vi "Fluigent_Pressure_Fluctuation_v3.vi"() -> ()   [LabVIEW 2020]
uses:
  <vilib>/DAQmx/read.llb/DAQmx Read (Analog 1D Wfm NChan NSamp).vi
  <userlib>/Fluigent/Fluigent MFCS/FluigentMFCS_Full.llb/MFCS_EZ Detect.vi
  <userlib>/Fluigent/Fluigent MFCS/FluigentMFCS_Full.llb/MFCS_EZ Initialization.vi
  <vilib>/DAQmx/create/channels.llb/DAQmx Create Channel (AI-Voltage-Basic).vi
  <vilib>/DAQmx/configure/timing.llb/DAQmx Timing (Sample Clock).vi
  <vilib>/DAQmx/miscellaneous.llb/DAQmx Fill In Error Info.vi
  <vilib>/Waveform/WDTOps.llb/WDT Get XY Value DBL.vi
  <userlib>/Fluigent/Fluigent MFCS/FluigentMFCS_Full.llb/MFCS_EZ Read All Channels Pressure.vi
  <userlib>/Fluigent/Fluigent MFCS/FluigentMFCS_Full.llb/MFCS_EZ Close.vi
  <vilib>/measure/NI_MABase.lvlib
panel:
  in  "Voltage Conversion Factor":dbl=100.0 caption="Voltage Conversion Factor (1 V = x mmHg)" format="%0.2f"
  out "Finished":bool
  out "Time Elapsed (Min)":cluster{dbl, dbl}(slide)={5.0, 0.0} scale=0.0..5.0 scale format="%#_2g"
  out "Dev1 Samples":i32
  out "Running":bool
  in  "sampling info":cluster{"Fs":dbl, "#s":dbl}
  in  "Fs":dbl
  in  "Time (min)":dbl(knob)=5.0 min=0.1 max=5.0 step=0.1 scale=0.0..5.0 scale format="%#_2g"
  in  "Index File Labels Fluigent System":string[](array[string])=["1000", "nobody", "test", "1", "1", "junk"]
  out "Analog File Name Fluigent":string="C:\\yurong\\141104_12_31_1104"
  in  "Path for files Fluigent System":path=path "C:/Users/kkg5246/Desktop/Research/Fluigent Recordings"
  out "Current Voltage (V)":dbl
  out "Current Pressure (mmHg)":dbl
  out "Actual Pressure":dbl[](graph)
  out "Theoretical Pressure Waveform":waveform(dbl)(graph)={"t0"=timestamp(15 s since 1904-01-01), "dt"=0.001, "Y"=[]}
  in  "Duty Cycle (%)":dbl=50.0 format="%0.2f"
  in  "Offset":dbl=250.0 format="%0.2p"
  in  "Reset Signal ?":bool
  in  "Signal Type":T1(ring)
  in  "Frequency (Hz)":dbl=5.0 format="%0.2p"
  in  "Amplitude (mmHg)":dbl=0.25 format="%0.2p"
  in  "Phase":dbl format="%0.2f"
  out "Phase out":dbl=180.0000000002135 format="%0.2f"
  in  "Stop":bool
  out "Waveform Chart":waveform(dbl)(graph)
  out "Pressure":dbl[](graph)=[0.00694105110600887]
  in  "physical channels":tag="Dev1/ai0"
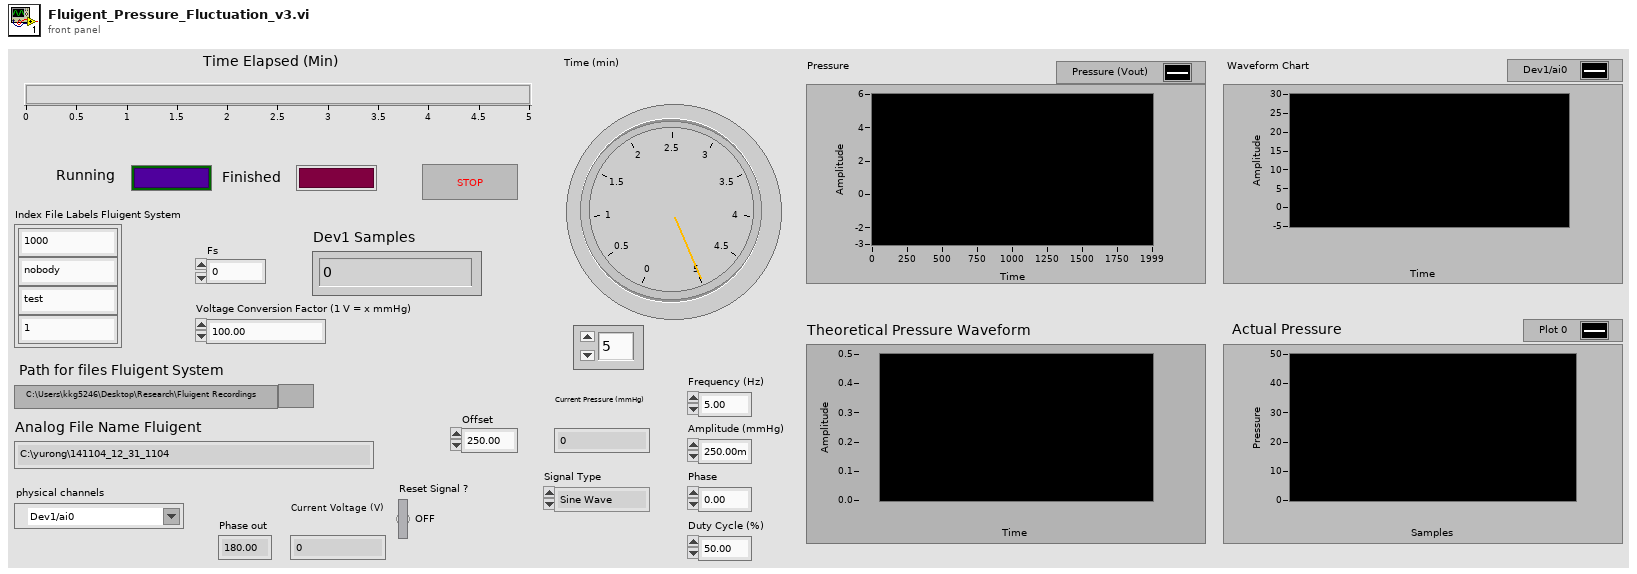
[diagram p1: front panel]
types:
  T1 = enum16{"Sine Wave", "Triangle Wave", "Square Wave", "Sawtooth Wave"}
  T2 = enum16{"open", "open or create", "create or replace", "create", "open (read-only)"}
  T3 = typedef "_EZmfcsSN.ctl" = u16
  T4 = typedef "_mfcs_EZ_handle.ctl" = u64
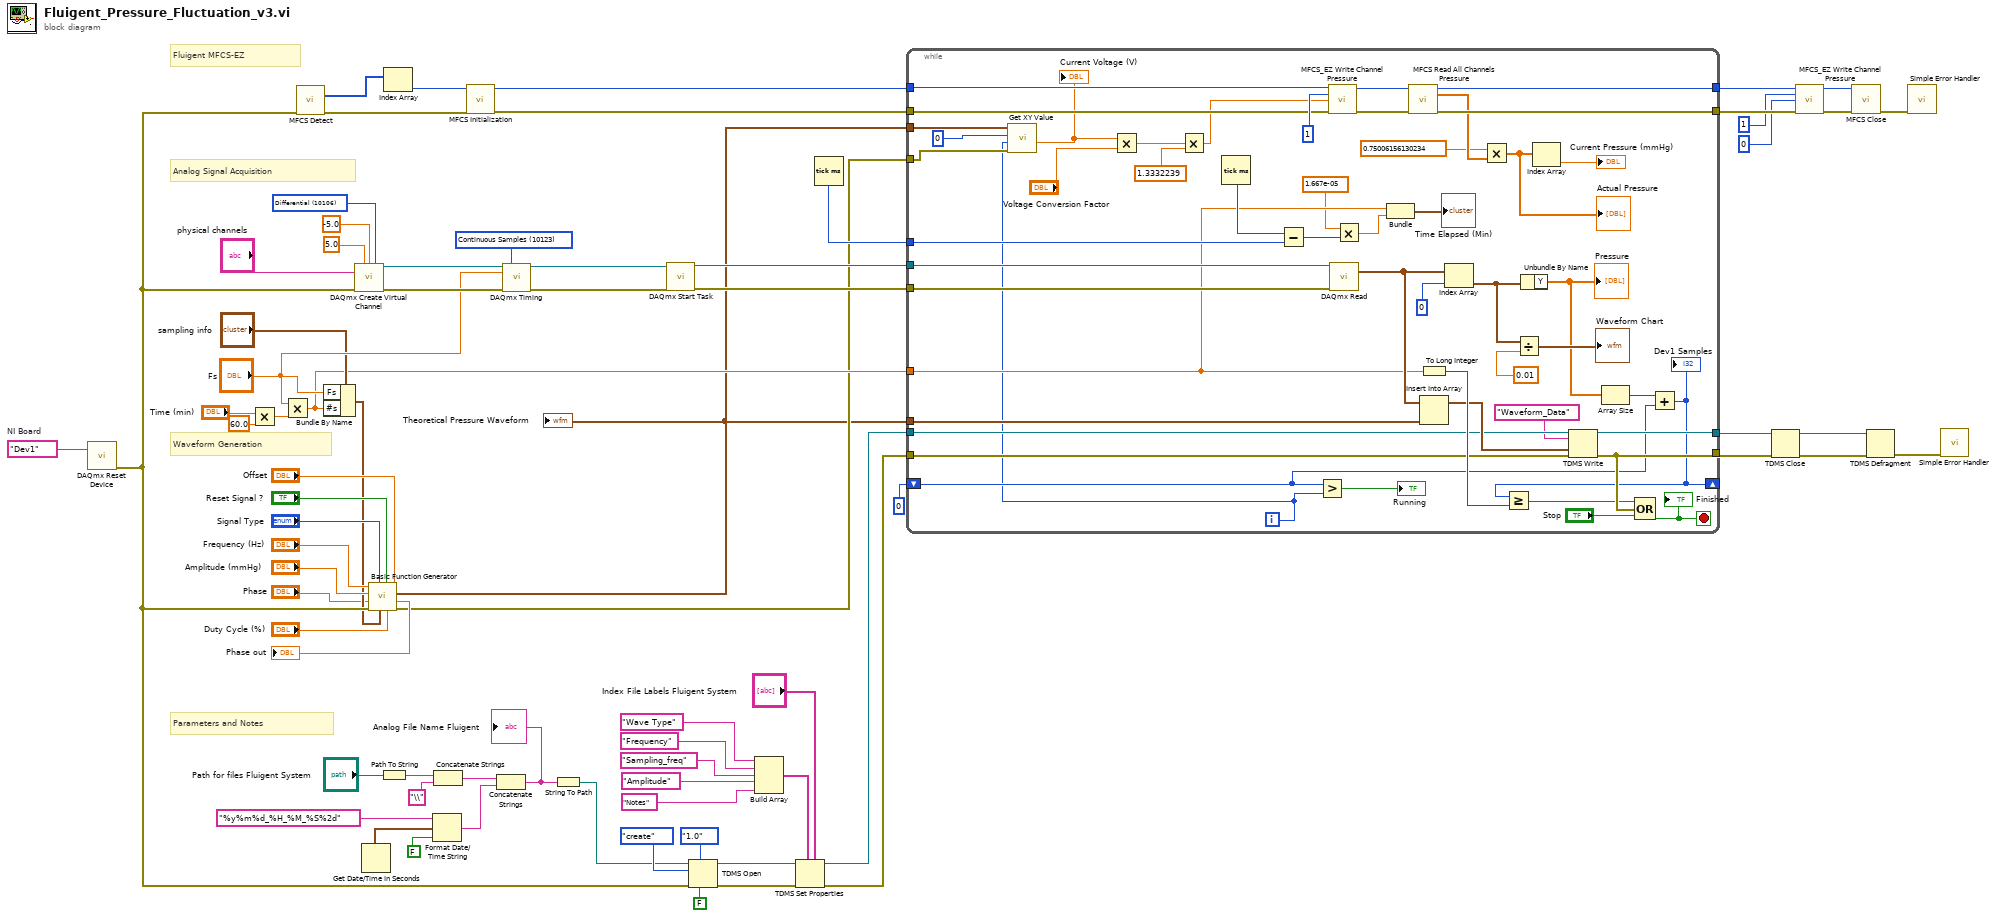
[diagram p0: block diagram]
diagram:
  w17 = tag "Dev1"  # NI Board
  w68 = 10106 items=["default"=-1, "RSE"=10083, "NRSE"=10078, "Differential"=10106, "Pseudodifferential"=12529] ("input terminal configuration")
  w72 = 10123 items=["Finite Samples"=10178, "Continuous Samples"=10123, "Hardware Timed Single Point"=12522] ("sample mode")
  # "Parameters and Notes"
  # "Waveform Generation"
  # "Analog Signal Acquisition"
  # "Fluigent MFCS-EZ"
  n1 = call <vilib>:"DAQmx Reset Device.vi"("device in"=w17) -> ("error out"=w16:errorcluster)  [unwired: 14 in]
  n2 = Multiply(x="Time (min)", y=60.0 ("minimum value")) -> (x*y=w5:dbl)
  n3 = Multiply(x="Fs", y=w5) -> (x*y=w9:dbl)
  n4 = call-poly <userlib>:"MFCS Detect.vi"("error in (no error)"=w16) -> ("[SN MFCS_EZ]"=w62:T3[], "error out"=w60:errorcluster)  [unwired: 13 in]
  n5 = Bundle By Name ("sampling info")(cluster="sampling info", "Fs"="Fs", "#s"=w9) -> (w15:cluster{"Fs":dbl, "#s":dbl})
  n6 = call-poly <vilib>:"DAQmx Create Virtual Channel.vi"("maximum value"=5.0, "minimum value"=-5.0, "input terminal configuration"=w68, "physical channels"="physical channels", "error in"=w16) -> ("task out"=w73:refnum<k21>, "error out"=w71:errorcluster)  [unwired: 4 in, 5 out]
  n7 = Get Date/Time In Seconds() -> (seconds since 1Jan1904=w48:timestamp)
  n8 = call <vilib>:"Basic Function Generator.vi"("offset"="Offset", "square wave duty cycle (%)"="Duty Cycle (%)", "reset signal"="Reset Signal ?", "sampling info"=w15, "signal type"="Signal Type", "error in (no error)"=w16, "phase"="Phase", "amplitude"="Amplitude (mmHg)", "frequency"="Frequency (Hz)") -> ("error out"=w2:errorcluster, "phase out"=→"Phase out":dbl, "signal out"=w1:waveform(dbl))
  "Theoretical Pressure Waveform" <- w1
  n9 = Path To String(path="Path for files Fluigent System") -> (string=w33:string)
  n10 = Index Array(array=w62) -> (element=w61:T3)  [unwired: 1 in]
  n11 = Format Date/Time String(time format string (%c)="%y%m%d_%H_%M_%S%2d", seconds (now)=w48, UTC format=FALSE) -> (date/time string=w45:string)
  n12 = Concatenate Strings(w33, "\\" ("string")) -> (w46:string)
  n13 = call-poly <userlib>:"MFCS Initialization.vi"("SN MFCS_EZ"=w61, "error in (no error)"=w60) -> ("MFCS_EZ_out"=w56:T4, "error out"=w55:errorcluster)  [unwired: 10 in, 2 out]
  n14 = Concatenate Strings(w46, w45) -> (w44:string)
  "Analog File Name Fluigent" <- w44
  n15 = call-poly <vilib>:"DAQmx Timing.vi"("task/channels in"=w73, "sample mode"=w72, "rate"="Fs", "error in"=w71) -> ("task out"=w66:refnum<k21>, "error out"=w65:errorcluster)  [unwired: 3 in, 7 out]
  n16 = String To Path(string=w44) -> (path=w40:path)
  n17 = call <vilib>:"DAQmx Start Task.vi"("task/channels in"=w66, "error in"=w65) -> ("task out"=w64:refnum<k21>, "error out"=w63:errorcluster)  [unwired: 12 out]
  n18 = TDMS Open(6:FALSE ("disable buffering? (T)"), 7:enum16{"1.0", "2.0"}."1.0" ("file format version (2.0)"), 8:w16, 10:T2."create" ("operation (0:open)"), 11:w40) -> (0:w39:errorcluster, 3:w31:refnum<k34>)  [unwired: 2 in]
  n19 = Build Array("Wave Type", "Frequency", "Sampling_freq", "Amplitude", "Notes") -> (w34:string[])
  n20 = TDMS Set Properties(5:"Index File Labels Fluigent System", 7:w34, 8:w39, 11:w31) -> (0:w29:errorcluster, 3:w26:refnum<k34>)  [unwired: 4 out]
  n21 = Tick Count (ms)() -> (millisecond timer value=w6:u32)
  n22 = while {
    tunnel: w64 -> [w119]
    tunnel: w63 -> [w114]
    tunnel: w56 -> [w115]
    tunnel: w55 -> [w113]
    tunnel: [w112] -> w54
    tunnel: [w111] -> w51
    tunnel: w29 -> [w94]
    tunnel: [w104] -> w27
    tunnel: w26 -> [w92]
    tunnel: w1 -> [w95]
    tunnel: [w106] -> w11
    shift-right: [w97] -> _
    shift-left: 0 -> [w98]
    tunnel: w9 -> [w86]
    tunnel: w6 -> [w88]
    tunnel: w2 -> [w79]
    tunnel: w1 -> [w78]
    i -> [w75]
    stop <- w83 stop-if-true
    n23 = call-poly <vilib>:"Get XY Value.vi"("error in (no error)"=w79, "Y position"=w75, "Y position format"=0, "waveform in"=w78) -> ("Y value"=w77:dbl)  [unwired: 3 in, 4 out]
    "Current Voltage (V)" <- w77
    n24 = Multiply(x=w77, y="Voltage Conversion Factor") -> (x*y=w82:dbl)
    n25 = Multiply(x=w82, y=1.3332239) -> (x*y=w76:dbl)
    n26 = Tick Count (ms)() -> (millisecond timer value=w89:u32)
    n27 = Subtract(x=w89, y=w88) -> (x-y=w85:u32)
    n28 = Greater?(x=w98, y=w75) -> (0:→"Running":bool)
    n29 = call <userlib>:"MFCS_EZ Write Channel Pressure.vi"("MFCS_EZ"=w115, "Channel Number (default=1)"=1, "Pressure (mBar)"=w76, "error in (no error)"=w113) -> ("MFCS_EZ out"=w117:T4, "error out"=w118:errorcluster)  [unwired: 10 in]
    n30 = call-poly <vilib>:"DAQmx Read.vi"("task/channels in"=w119, "error in"=w114) -> ("data"=w96:waveform(dbl)[])  [unwired: 1 in, 12 out]
    n31 = Multiply(x=1.667e-05, y=w85) -> (x*y=w90:dbl)
    n32 = Bundle(w86, w90) -> (→"Time Elapsed (Min)":cluster{dbl, dbl})  [unwired: 1 in]
    n33 = call-poly <userlib>:"MFCS Read All Channels Pressure.vi"("MFCS_EZ"=w117, "error in (no error)"=w118) -> ("MFCS_EZ out"=w111:T4, "All Channels Pressure"=w110:dbl[], "error out"=w112:errorcluster)  [unwired: 11 in]
    n34 = To Long Integer(number=w86) -> (32bit integer=w102:i32)
    n35 = Insert Into Array(array=w96, new element=w95) -> (w93:waveform(dbl)[])  [unwired: 1 in]
    n36 = Index Array "Index Array"(array=w96, index=0 ("index (row)")) -> (element=w120:waveform(dbl))
    n37 = Multiply(x=0.75006156130234, y=w110) -> (x*y=w108:dbl[])
    "Actual Pressure" <- w108
    n38 = Divide(x=w120, y=0.01) -> (x/y=→"Waveform Chart":waveform(dbl))
    n39 = Unbundle By Name(w120) -> ("Y"=w100:dbl[])
    "Pressure" <- w100
    n40 = Index Array(array=w108) -> (element=→"Current Pressure (mmHg)":dbl)  [unwired: 1 in]
    n41 = TDMS Write(0:w92, 5:"Waveform_Data" ("string"), 9:w93, 11:w94) -> (4:w106:refnum<k34>, 15:w104:errorcluster)  [unwired: 2 in, 2 out]
    n42 = Array Size(array=w100) -> (size(s)=w99:i32)
    n43 = Add(x=w99, y=w98) -> (x+y=w97:i32)
    "Dev1 Samples" <- w97
    n44 = Greater Or Equal?(x=w97, y=w102) -> (x >= y?=w101:bool)
    n45 = Compound Arithmetic op=OR(w101, w104, "Stop") -> (w83:bool)
    "Finished" <- w83
  }
  n46 = TDMS Close(8:w27, 11:w11) -> (0:w28:errorcluster, 3:w7:path)
  n47 = call <userlib>:"MFCS_EZ Write Channel Pressure.vi"("MFCS_EZ"=w51, "Channel Number (default=1)"=1, "Pressure (mBar)"=0, "error in (no error)"=w54) -> ("MFCS_EZ out"=w57:T4, "error out"=w58:errorcluster)  [unwired: 10 in]
  n48 = call-poly <userlib>:"MFCS Close.vi"("MFCS_EZ"=w57, "error in (no error)"=w58) -> ("error out"=w59:errorcluster)  [unwired: 13 in]
  n49 = TDMS Defragment(4:w28, 7:w7) -> (0:w8:errorcluster)
  n50 = call <vilib>:"Simple Error Handler.vi"("error in (no error)"=w59) -> ()  [unwired: 4 in, 5 out]
  n51 = call <vilib>:"Simple Error Handler.vi"("error in (no error)"=w8) -> ()  [unwired: 4 in, 5 out]
